vi "DelayTables.vi"() -> ()   [LabVIEW 2022 SP3]
uses:
  <vilib>/Analysis/NI_AALPro.lvlib
  <vilib>/Analysis/NI_AALBase.lvlib
  <vilib>/Analysis/2dsp.llb/1D Cross Correlation (DBL).vi
  <vilib>/Utility/file.llb/Write Delimited Spreadsheet (DBL).vi
  ViewData/-ReadEye/ScaleMethod.ctl
  -AnnularRoutines/ArrayGeometry.ctl
  -AnnularRoutines/TransGeometry.ctl
panel:
  in  "Filter Prams":T1={"low cutoff"=5, "order"=81, "high cutoff"=35}
  in  "Type of Mean":u16(ring) items=["Mean from lines", "Mean just lines", "Poly Mean", "No mean", "Filter"]
  in  "Trans Geometry (mm) out":T2={"Transducer"=0, "Geo Focus"=12.0, "a (radius)"=3.0, "# of rings"=5, "kerf space "=0.1, "Center Freq"=12.0} {"Transducer" items=["6D 12R 40 MHz"=0, "10D 31R 20 MHz"=1, "10D 23R 20 MHz"=2, "6D 23R 40 MHz"=3, "4.5D 10.7R 40 MHz"=4, "9D 23.5R 20 MHz"=5, "9D 25.8R 20MHz"=6, "Enter"=99]}
  in  "index (page)":i32
  in  "d":u8
  out "Blow up of yellow Line 3":dbl[][](graph)
  in  "Case Constant\n(See Context Help)":bool
  out "Waveform Graph":dbl[][](graph)
  in  "Tab Control":enum32{"Page 1", "Page 2", "Page 3"}(tab)
  out "rel set of 6":i32[][](array[numeric])
  in  "Rings mm 2":sgl[](array[numeric])=[0.0, 1.32, 1.42, 1.9, 2.0, 2.36, 2.46, 2.75, 2.85, 3.1]
  out "data delays stacked":i32[][](array[numeric])
  out "rel set of 5":i32[][](array[numeric])
  in  "furthest first?":bool
  out "data delays":i32[][][](array[numeric])
  out "Array":dbl[][](array[numeric]) format="%.2f"
  out "delays abs":dbl[][][](array[numeric]) format="%.2f"
  in  "sampling rate":dbl=1e-09
  in  "focus mm":dbl=12.0
  in  "Rings mm":sgl[](array[numeric])=[0.0, 1.22, 1.32, 1.8, 1.9, 2.26, 2.36, 2.65, 2.75, 3.0]
  in  "focus locations":sgl[](array[numeric])=[9.0, 10.2, 11.0, 12.0, 13.0, 14.0, 15.0]
  in  "sound speed mm/s":dbl=1485000.0
  out "delays":sgl[][](array[numeric]) format="%#_2g"
  in  "delay offset":sgl
  in  "Corr(T)/Thresh(F)":bool
  out "Wire Locations mm":dbl[](array[numeric]) format="%0.2f"
  in  "View Header?":bool
  in  "Axis scaling":bool=TRUE
  out "Scan line peaks":dbl[](array[numeric]) format="%0.2f"
  out "Wire Locations RF":dbl[](array[numeric]) format="%0.2f"
  out "Blow up of yellow Line 2":sgl[](graph)
  in  "new file path":path=path "F:/PVDFXducer/FiveRing/5Ring5/83micH/Wire Phantom/25 micron/WireAugd 1to1.eye"
  out "Blow up of yellow Line":dbl[][](graph)
  out "Raw data":dbl[][](graph)
  in  "Display mode":T4=enum."Log Grey Scale"
  in  "threshold":dbl=20.0 format="%0.2f"
  in  "width":i32=10 min=3
  out "Waveform Graph 2":dbl[][](graph)
  out "Intensity Graph":dbl[][](graph)
  # "time steps to shift relative to zero"
  # "rings"
  # "distances"
  # "Each plane is delays for single focal distance. Negative means subtract zeroes."
  # "receive"
  # "transmit"
  # "relative delays to ring one. Each row is a different focal depth"
  # "Delays relative to ring 1. Starting at furthest ring"
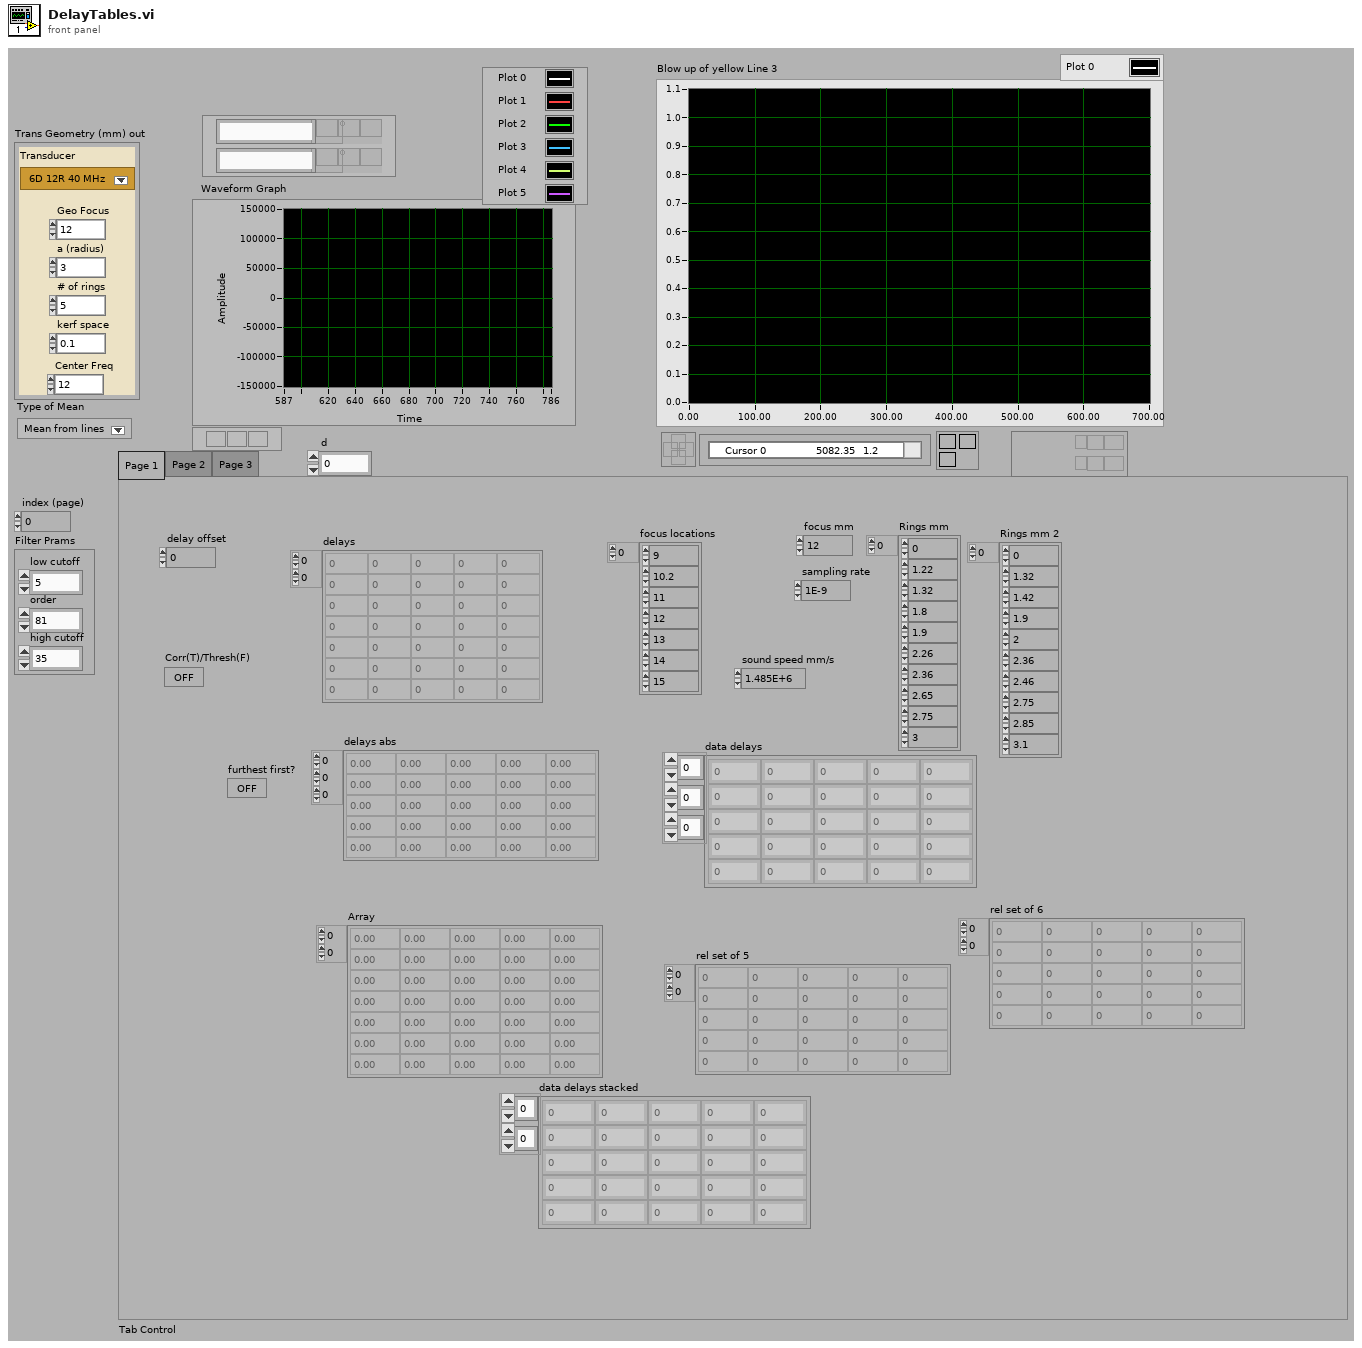
[diagram p1: front panel]
types:
  T1 = cluster{"low cutoff":i32, "order":i32, "high cutoff":i32}
  T2 = typedef "TransGeometry.ctl" = cluster{"Transducer":T3, "Geo Focus":dbl, "a (radius)":dbl, "# of rings":i32, "kerf space ":dbl, "Center Freq":dbl}
  T3 = typedef "ArrayGeometry.ctl" = u16
  T4 = typedef "ScaleMethod.ctl" = enum16{"Linear Abs Grey", "Log Grey Scale", "Linear Color Scale", "dB Scale", "Verasonics Doppler"}
  T5 = typedef "Header.ctl" = cluster{"header info":cluster{"Header":string, "Head length":i16}, "A/D info":cluster{"# rf points per line":u16, "# lines per scan":u16, "sample rate MHz":u16, "# A/D bits":i16, "# bytes per A/D":u16, "TGC Flag":u16, "A/D Type":string}, "Tranducer Info":cluster{"bandwidth":sgl, "center freq":sgl, "start freq":sgl, "ID":i32}, "Scan Info":cluster{"delay":sgl, "pivot distance":sgl, "sector scan angle":sgl, "operator":string, "Scan Mode":string, "location":string}, "Time/Date Info":cluster{"date":string, "time":string}, "RF Info":cluster{"RF file name":string, "RF file att":string, "RF cal file name":string, "RF cal file att":string}, "Patient Info":cluster{"ID":string, "extended ID":string, "age":u16, "sex":string, "previously\nscanned":string, "PSA":sgl, "LOS":u8, "Ethnicty 2":u8, "Race":u8}, "Tissue Type":cluster{"organ":i16, "disease type":i16, "disease location":i16, "IQ_pts":u16, "RcvBuffer":u8, "RcvFrame":u16, "IQBuff":u8, "IQFrame":u16, "IQPage":u8}, "Votage scaling":cluster{"Digitizer (dB)":sgl, "Gain (dB)":sgl, "Atten (dB)":sgl}, "Comment":string, "Misc Info":cluster{"avg num":u16, "c speed":i16, "Div By or SF zones":i16, "XMIT CHS":u8, "RCV CHS":u8, "Xmit angle":sgl}, "Therapy Parameters":cluster{"Theraputic Freq (MHz)":sgl, "Time on (s)":sgl, "Therapy amplitude (mV)":sgl, "Lines Before":u16, "Lines After":u16}, "Scan Settings":cluster{"Energy (uJ or V)":u8, "Damp (Ohm) or Fc":u8, "HP Filt (KHz)":u8, "LP Filt (MHz)":u8, "Gain (db)":u8, "prf (kHz)":sgl, "Distance between\nscan lines (um)":u16, "Distance between\nscan planes (um)":u16, "Scan line gap (um)":sgl, "Scan plane gap (um)":sgl}, "Compression Parameters":cluster{"F1 (MHz)":sgl, "F2 (MHz)":sgl, "% taper":sgl, "duration":sgl}, "Patient Info Xtra":cluster{"First Name":string, "Last Name":string, "Notes":string}, "ROI Box":u16[]}
  T6 = cluster{"Energy (uJ) or V":u8, "Damp (Ohm) or Fc":u8, "HP Filt(KHz) ":u8, "LP Filt (MHz)":u8, "Gain (db)":u8, "prf (kHz)":sgl, "Distance between\nscan lines (mm)":u16, "Distance between\nscan planes (mm)":u16, "Scan line gap (um)":sgl, "Scan plane gap (um)":sgl}
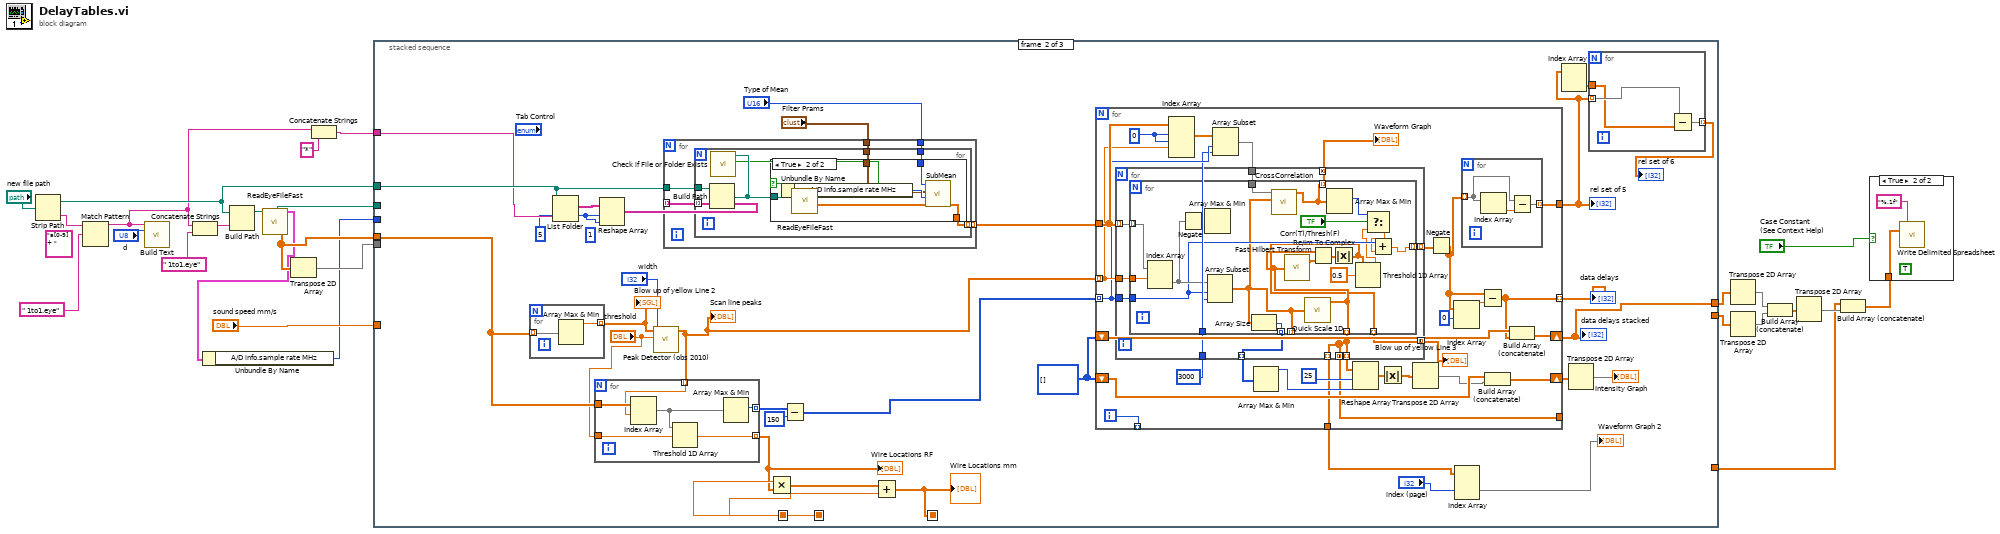
[diagram p0: block diagram]
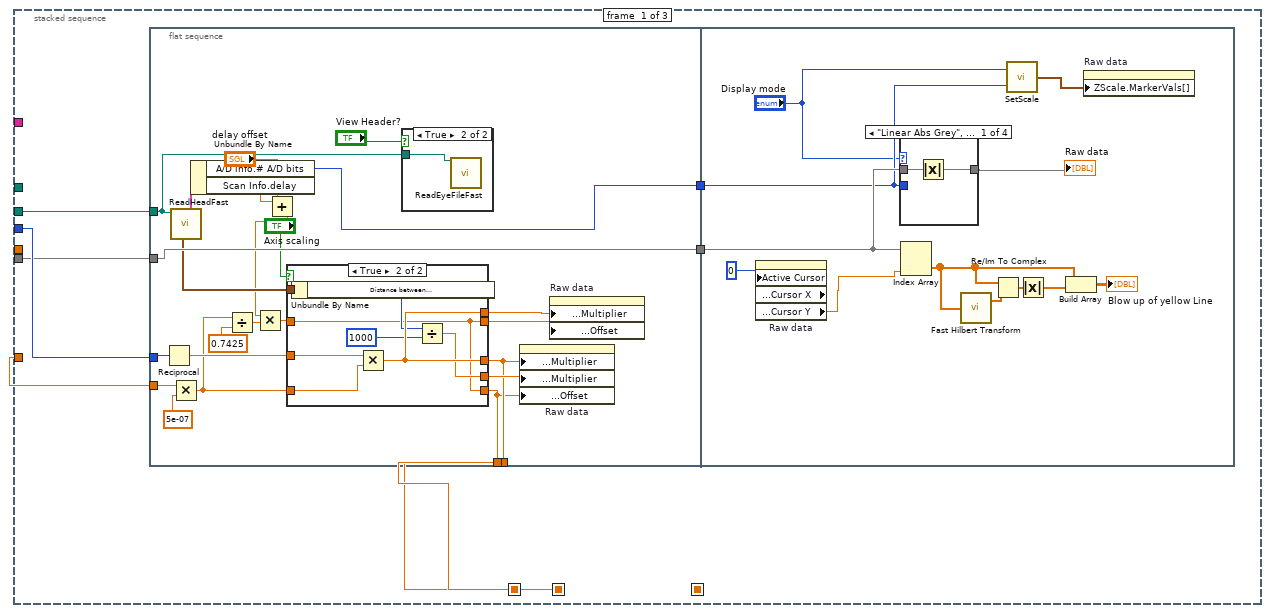
[diagram p3: hidden frame]
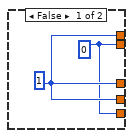
[diagram p5: hidden frame]
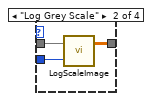
[diagram p6: hidden frame]
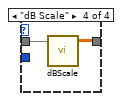
[diagram p8: hidden frame]
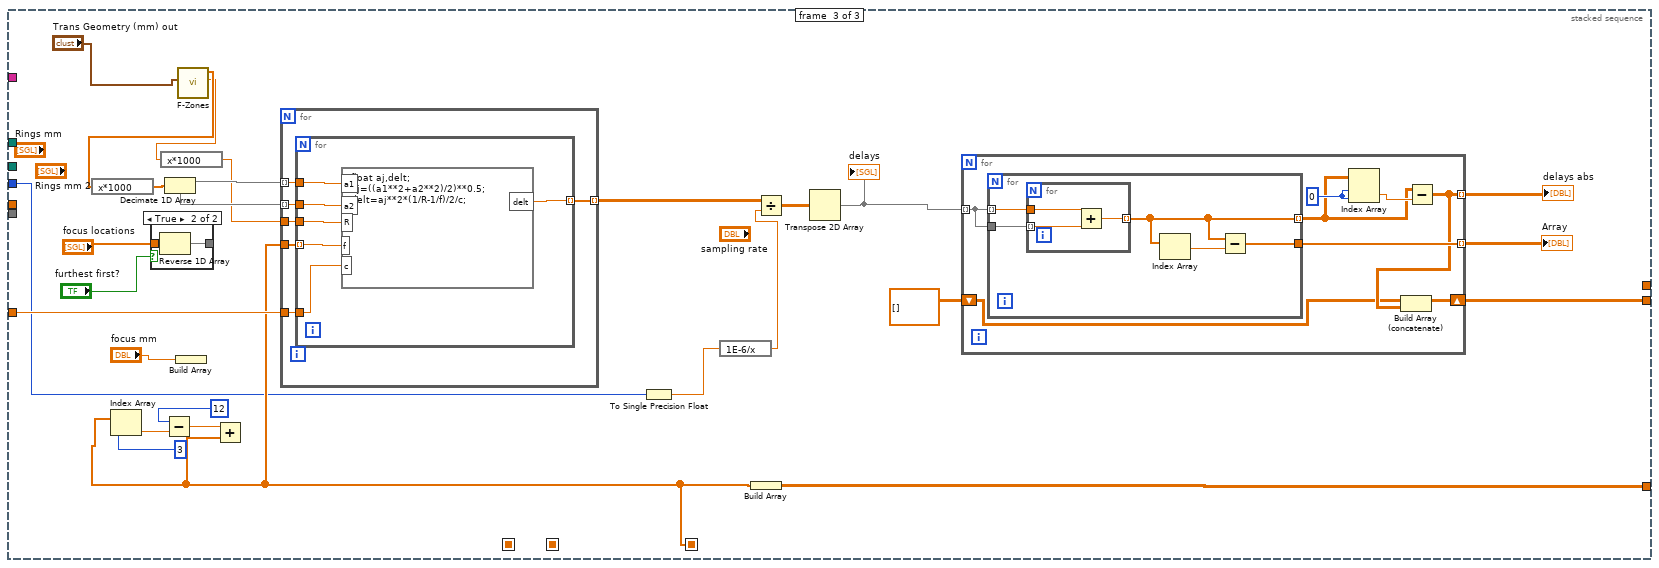
[diagram p10: hidden frame]
diagram:
  (unwired) "a[0-9]+ " ("regular expression")
  n1 = Strip Path(path="new file path") -> (stripped path=w8:path, name=w11:string)
  n2 = Match Pattern(string=w11, regular expression=" 1to1.eye" ("string")) -> (before substring=w1:string)  [unwired: 1 in, 3 out]
  n3 = call "Build Text"("Beginning Text"=w1, "d"="d") -> ()  [unwired: 12 in, 2 out]
  n4 = Concatenate Strings(w1, " 1to1.eye" ("string")) -> (w10:string)
  n5 = Build Path(base path=w8, name or relative path=w10) -> (appended path=w9:path)
  n6 = call "ReadEyeFileFast.vi"("new file path"=w9) -> ("new path out"=w26:path, "2-D data array"=w14:sgl[][], "Header In"=w4:T5)  [unwired: 13 in, 3 out]
  n7 = Unbundle By Name(w4) -> ("A/D info.sample rate MHz"=w3:u16)
  n8 = Transpose 2D Array(2D array=w14) -> (transposed array=w15:sgl[][])
  n9 = Concatenate Strings(w1, "*" ("string")) -> (w5:string)
  n10 = stacked-sequence {
    seq-local: [w30 _ _] -> [_ w116 _]
    seq-local: [w29 _ _] -> [_ w117 _]
    seq-local: [_ w111 _] -> [_ _ w223]
    tunnel: w15 -> [w27 _ _]
    tunnel: w26 -> [w33 _ _]
    tunnel: w3 -> [w32 _ w216]
    tunnel: "sound speed mm/s" -> [w31 _ w233]
    tunnel: [_ _ w227] -> w22
    tunnel: [_ w113 _] -> w23
    tunnel: [_ _ w224] -> w16
    tunnel: w14 -> [_ w109 _]
    tunnel: w8 -> [_ w101 _]
    tunnel: w5 -> [_ w100 _]
    frame #0 {
      n11 = flat-sequence {
        tunnel: w27 -> [w57]
        tunnel: [w57] -> w34
        tunnel: w33 -> [w46]
        tunnel: w32 -> [w52]
        tunnel: w31 -> [w48]
        tunnel: [w45] -> w29
        tunnel: [w44] -> w30
        tunnel: [w38] -> w28
        tunnel: w34 -> [w74]
        tunnel: w28 -> [w71]
        frame #0 {
          n12 = Reciprocal(x=w52) -> (1/x=w51:dbl)
          n13 = call "ReadHeadFast.vi"("new file path"=w46) -> ("Header In"=w39:T5, "Scan Settings (Pulser and Scaping)"=w53:T6)  [unwired: 7 in, 2 out]
          n14 = Multiply(x=w48, y=5e-07) -> (x*y=w42:dbl)
          n15 = Unbundle By Name(w39) -> ("A/D info.# A/D bits"=w38:i16, "Scan Info.delay"=w37:sgl)
          n16 = Divide(x=w42, y=0.7425) -> (x/y=w41:dbl)
          n17 = Add(x=w37, y="delay offset") -> (x+y=w36:sgl)
          n18 = Multiply(x=w36, y=w41) -> (x*y=w40:dbl)
          n19 = case shown="True" "Axis scaling" {
            tunnel: [w60 w68] -> w45
            tunnel: [w60 w68] -> w54
            tunnel: w53 -> [_ w67]
            tunnel: [w60 w64] -> w55
            tunnel: [w59 w63] -> w56
            tunnel: w40 -> [_ w63]
            tunnel: [w59 w63] -> w44
            tunnel: w51 -> [_ w62]
            tunnel: w42 -> [_ w61]
            frame False {
              w59 = 0
              w60 = 1
            }
            frame True {
              n20 = Unbundle By Name(w67) -> ("Distance between\nscan lines (mm)"=w66:u16)
              n21 = Multiply(x=w62, y=w61) -> (x*y=w68:dbl)
              n22 = Divide(x=w66, y=1000) -> (x/y=w64:dbl)
            }
          }
          n23 = case shown="True" "View Header?" {
            tunnel: w46 -> [_ w58]
            frame False {
            }
            frame True {
              n24 = call "ReadEyeFileFast.vi"("new file path"=w58) -> ()  [unwired: 13 in, 6 out]
            }
          }
          n25 = property on="Raw data" class="IntGraph (strict)"("X Scale.Offset and Multiplier:Multiplier"=w45, "Y Scale.Offset and Multiplier:Multiplier"=w55, "X Scale.Offset and Multiplier:Offset"=w44) -> ()  [unwired: 2 in, 2 out]
          n26 = property on="Raw data" class="IntGraph (strict)"("X Scale.Offset and Multiplier:Multiplier"=w54, "X Scale.Offset and Multiplier:Offset"=w56) -> ()  [unwired: 2 in, 2 out]
        }
        frame #1 {
          n27 = property on="Raw data" class="IntGraph (strict)" props=["Active Cursor", "Cursor", "Cursor Position:Cursor X", "Cursor", "Cursor Position:Cursor Y"]("Active Cursor"=u32 0 ("Write Attribute")) -> ("Cursor.Cursor Position:Cursor Y"=w73:dbl)  [unwired: 2 in, 3 out]
          n28 = case shown="\"Linear Abs Grey\", Default" "Display mode" {
            tunnel: [w81 w85 w86 w87] -> w69
            tunnel: w74 -> [w82 w84 w86 w88]
            tunnel: w71 -> [_ w83 _ _]
            frame "Linear Abs Grey", Default {
              n29 = Absolute Value(x=w82) -> (abs(x)=w81:sgl[][])
            }
            frame "Log Grey Scale" {
              n30 = call "LogScaleImage.vi"("A/D bits"=w83, "input array"=w84) -> ("log scale image"=w85:dbl[][])  [unwired: 1 out]
            }
            frame "Linear Color Scale" {
            }
            frame "dB Scale" {
              n31 = call "dBScale.vi"("Data In"=w88) -> ("Data Out"=w87:dbl[][])  [unwired: 4 in]
            }
          }
          "Raw data" <- w69
          n32 = Index Array(array=w74, index (col)=w73) -> (element=w80:sgl[])  [unwired: 1 in]
          n33 = call <vilib>:"Fast Hilbert Transform.vi"("X"=w80) -> ("Hilbert{X}"=w77:dbl[])  [unwired: 1 out]
          n34 = Re/Im To Complex(1:w77, 2:w80) -> (0:w76:cdb[])
          n35 = call "SetScale.vi"("# A/D bits"=w71, "Display mode"="Display mode") -> ("Array"=w72:cluster{dbl, u32}[])
          n36 = Absolute Value(x=w76) -> (abs(x)=w79:dbl[])
          n37 = Build Array(w80, w79) -> (→"Blow up of yellow Line":dbl[][])
          n38 = property on="Raw data" class="IntGraph (strict)"("ZScale.MarkerVals[]"=w72) -> ()  [unwired: 2 in, 2 out]
        }
      }
    }
    frame #1 {
      (unwired) 1
      w99 = 5
      w107 = i32[][] []
      n39 = for {
        tunnel: w109 -> [w212] mode=indexing
        tunnel: [w211] -> w112 mode=indexing
        n40 = Array Max & Min(array=w212) -> (max value=w211:sgl)  [unwired: 3 out]
      }
      "Blow up of yellow Line 2" <- w112
      n41 = List Folder(path=w101, pattern=w100) -> (filenames=w105:string[])  [unwired: 1 in, 4 out]
      n42 = Reshape Array(w105, w99, w99) -> (w106:string[][])
      n43 = call <vilib>:"Peak Detector (obs 2010).vi"("width"="width", "threshold"="threshold", "X"=w112) -> ("Locations"=w110:dbl[])  [unwired: 4 in, 4 out]
      "Scan line peaks" <- w110
      n44 = for {
        tunnel: [w209] -> w114 mode=indexing
        tunnel: w109 -> [w210]
        tunnel: w110 -> [w206] mode=indexing
        tunnel: [w207] -> w115 mode=indexing
        tunnel: "threshold" -> [w205]
        n45 = Index Array(array=w210, index (row)=w206) -> (element=w208:sgl[])  [unwired: 1 in]
        n46 = Threshold 1D Array(2:w205, 3:w208) -> (0:w207:sgl)  [unwired: 1 out]
        n47 = Array Max & Min(array=w208) -> (max index (indices)=w209:i32)  [unwired: 3 out]
      }
      "Wire Locations RF" <- w115
      n48 = for {
        tunnel: [w128] -> w104 mode=indexing
        tunnel: w106 -> [w127] mode=indexing
        tunnel: w101 -> [w126]
        tunnel: "Type of Mean" -> [w125]
        tunnel: "Filter Prams" -> [w124]
        n49 = for {
          tunnel: [w131] -> w128 mode=indexing
          tunnel: w127 -> [w135] mode=indexing
          tunnel: w126 -> [w134]
          tunnel: w125 -> [w130]
          tunnel: w124 -> [w129]
          n50 = Build Path(base path=w134, name or relative path=w135) -> (appended path=w133:path)
          n51 = call <vilib>:"Check if File or Folder Exists.vi"("path"=w133) -> ("file or folder exists?"=w132:bool)  [unwired: 8 in, 2 out]
          n52 = case shown="True" w132 {
            tunnel: w133 -> [_ w142]
            tunnel: [_ w140] -> w131
            tunnel: w130 -> [_ w139]
            tunnel: w129 -> [_ w136]
            frame False {
            }
            frame True {
              n53 = call "ReadEyeFileFast.vi"("new file path"=w142) -> ("2-D data array"=w141:sgl[][], "Header In"=w138:T5)  [unwired: 13 in, 4 out]
              n54 = Unbundle By Name(w138) -> ("A/D info.sample rate MHz"=w137:u16)
              n55 = call "SubMean.vi"("Scan Data In"=w141, "Samp Rate (MHz)"=w137, "Filter Prams"=w136, "Type of Mean"=w139) -> ("Array"=w140:dbl[][])  [unwired: 1 in, 2 out]
            }
          }
        }
      }
      n56 = Multiply(x=w117, y=w115) -> (x*y=w118:dbl[])
      n57 = Subtract(x=w114, y=150) -> (x-y=w119:i32[])
      n58 = Add(x=w118, y=w116) -> (x+y=w111:dbl[])
      "Wire Locations mm" <- w111
      n59 = for {
        tunnel: w110 -> [w150] mode=indexing
        tunnel: [w162] -> w108 mode=indexing
        tunnel: w119 -> [w149] mode=indexing
        shift-right: [w166] -> w103
        shift-left: w107 -> [w161]
        shift-right: [w164] -> w113
        shift-left: w107 -> [w163]
        tunnel: w104 -> [w157]
        tunnel: [w158] -> w95
        tunnel: [w152] -> _ mode=indexing
        tunnel: [w145] -> _
        tunnel: [w143] -> w98
        i -> [w152]
        w151 = 0
        w148 = 3000
        w170 = 0
        n60 = Index Array(array=w157, index (dim 0)=w151, index (dim 1)=w151, index (dim 2)=w150) -> (element=w155:dbl[])  [unwired: 1 in]
        n61 = Array Subset(array=w155, index=w149, length=w148) -> (w156:dbl[])
        n62 = for {
          tunnel: [w175] -> w171 mode=indexing
          tunnel: [w184] -> w168 mode=indexing
          tunnel: w150 -> [w183]
          tunnel: w148 -> [w182]
          tunnel: w149 -> [w181]
          tunnel: w157 -> [w180] mode=indexing
          tunnel: w156 -> [w179]
          tunnel: [w178] -> w154 mode=indexing
          tunnel: [w177] -> w147 mode=concatenating
          tunnel: [w175] -> w145 mode=concatenating
          tunnel: [w176] -> w144 mode=concatenating
          tunnel: [w175] -> w143 mode=indexing
          n63 = for {
            tunnel: [w194] -> w184 mode=indexing
            tunnel: [w190] -> w175 mode=indexing
            tunnel: w183 -> [w197]
            tunnel: w182 -> [w195]
            tunnel: w181 -> [w196]
            tunnel: w180 -> [w201] mode=indexing
            tunnel: w179 -> [w199]
            tunnel: [w198] -> w178 mode=indexing
            tunnel: [w189] -> w177 mode=indexing
            tunnel: [w193] -> _ mode=indexing
            tunnel: [w191] -> w176 mode=indexing
            n64 = Index Array(array=w201, index (row)=w197) -> (element=w200:dbl[])  [unwired: 1 in]
            n65 = Negate(x=w200) -> (-x=w192:dbl[])
            n66 = Array Max & Min(array=w192) -> ()  [unwired: 4 out]
            n67 = Array Subset(array=w200, index=w196, length=w195) -> (w193:dbl[])
            n68 = Array Size(array=w193) -> (size(s)=w198:i32)
            n69 = call-poly <vilib>:"CrossCorrelation.vi"("Y"=w193, "X"=w199) -> ("Rxy"=w191:dbl[])  [unwired: 2 in, 7 out]
            n70 = call <vilib>:"Quick Scale 1D.vi"("X"=w193) -> ("Y[i]=X[i]/Max|X|"=w190:dbl[])  [unwired: 2 out]
            n71 = call <vilib>:"Fast Hilbert Transform.vi"("X"=w190) -> ("Hilbert{X}"=w202:dbl[])  [unwired: 1 out]
            n72 = Re/Im To Complex(1:w202, 2:w190) -> (0:w203:cdb[])
            n73 = Array Max & Min(array=w191) -> (max index (indices)=w188:i32)  [unwired: 3 out]
            n74 = Absolute Value(x=w203) -> (abs(x)=w189:dbl[])
            n75 = Threshold 1D Array(2:0.5, 3:w189) -> (0:w187:dbl)  [unwired: 1 out]
            n76 = Select(t=w188, s="Corr(T)/Thresh(F)", f=w187) -> (s? t:f=w186:dbl)
            n77 = Add(x=w196, y=w186) -> (x+y=w194:dbl)
          }
        }
        "Blow up of yellow Line 3" <- w147
        "Waveform Graph" <- w144
        n78 = Array Max & Min(array=w154) -> (max value=w153:i32)  [unwired: 3 out]
        n79 = Reshape Array(w171, 25, w153) -> (w146:dbl[][])
        n80 = Absolute Value(x=w146) -> (abs(x)=w165:dbl[][])
        n81 = Transpose 2D Array(2D array=w165) -> (transposed array=w160:dbl[][])
        n82 = Negate(x=w168) -> (-x=w159:dbl[][])
        n83 = Index Array(array=w159, index (row)=w170, index (col)=w170) -> (element=w169:dbl)
        n84 = for {
          tunnel: w159 -> [w173] mode=indexing
          tunnel: [w172] -> w158 mode=indexing
          n85 = Index Array(array=w173) -> (element=w174:dbl)  [unwired: 1 in]
          n86 = Subtract(x=w173, y=w174) -> (x-y=w172:dbl[])
        }
        n87 = Subtract(x=w159, y=w169) -> (x-y=w162:dbl[][])
        n88 = Build Array (concatenate)(w161, w160) -> (w166:dbl[][])
        n89 = Build Array (concatenate)(w163, w162) -> (w164:dbl[][])
      }
      "data delays" <- w108
      "data delays stacked" <- w113
      "rel set of 5" <- w95
      n90 = Index Array(array=w98, index (dim 1)="index (page)") -> (element=→"Waveform Graph 2":dbl[][])  [unwired: 2 in]
      n91 = Index Array(array=w95) -> (element=w94:dbl[])  [unwired: 2 in]
      n92 = Transpose 2D Array(2D array=w103) -> (transposed array=→"Intensity Graph":dbl[][])
      n93 = for {
        tunnel: w95 -> [w123] mode=indexing
        tunnel: [w122] -> w93 mode=indexing
        tunnel: w94 -> [w121]
        n94 = Subtract(x=w123, y=w121) -> (x-y=w122:dbl[])
      }
      "rel set of 6" <- w93
    }
    frame #2 {
      n95 = Index Array(array=w223, index=3) -> (element=w229:dbl)
      n96 = case shown="True" "furthest first?" {
        tunnel: "focus locations" -> [w240 w242]
        tunnel: [w240 w241] -> _
        frame False {
        }
        frame True {
          n97 = Reverse 1D Array(array=w242) -> (reversed array=w241:sgl[])
        }
      }
      n98 = Subtract(x=12, y=w229) -> (x-y=w231:dbl)
      n99 = Build Array("focus mm") -> ()  [unwired: 1 out]
      n100 = call "F-Zones.vi"("Trans Geometry (mm)"="Trans Geometry (mm) out") -> ("ROC (m)"=w220:dbl, "annuli rad (m)"=w222:dbl[])  [unwired: 7 in, 2 out]
      n101 = expression code="x*1000"(w222) -> (w221:dbl[])
      n102 = expression code="x*1000"(w220) -> (w219:dbl)
      n103 = Decimate 1D Array(w221) -> (w238:dbl[], w237:dbl[])
      n104 = Add(x=w231, y=w223) -> ()  [unwired: 1 out]
      n105 = for {
        tunnel: w233 -> [w248]
        tunnel: w223 -> [w247]
        tunnel: w238 -> [w246] mode=indexing
        tunnel: w237 -> [w245] mode=indexing
        tunnel: [w244] -> w236 mode=indexing
        tunnel: w219 -> [w243]
        n106 = for {
          tunnel: w247 -> [w254] mode=indexing
          tunnel: w248 -> [w253]
          tunnel: w246 -> [w252]
          tunnel: w245 -> [w251]
          tunnel: [w250] -> w244 mode=indexing
          tunnel: w243 -> [w249]
          n107 = formula code="float aj,delt;\naj=((a1**2+a2**2)/2)**0.5;\ndelt=aj**2*(1/R-1/f)/2/c;"("a1"=w252, "a2"=w251, "f"=w254, "c"=w253, "R"=w249) -> ("delt"=w250:dbl)
        }
      }
      n108 = To Single Precision Float(number=w216) -> (single precision float=w215:sgl)
      n109 = expression code="1E-6/x"(w215) -> (w213:sgl)
      n110 = Build Array(w223) -> (w224:dbl[][])
      n111 = Divide(x=w236, y=w213) -> (x/y=w214:dbl[][])
      n112 = Transpose 2D Array(2D array=w214) -> (transposed array=w235:dbl[][])
      "delays" <- w235
      n113 = for {
        tunnel: w235 -> [w262] mode=indexing
        tunnel: [w257] -> w226 mode=indexing
        tunnel: [w261] -> w225 mode=indexing
        shift-right: [w255] -> w227
        shift-left: dbl[][] [] -> [w256]
        w260 = 0
        n114 = for {
          tunnel: w262 -> [w266] mode=indexing
          tunnel: w262 -> [w267]
          tunnel: [w263] -> w258 mode=indexing
          tunnel: [w264] -> w261
          n115 = for {
            tunnel: w267 -> [w270] mode=indexing
            tunnel: w266 -> [w269]
            tunnel: [w268] -> w263 mode=indexing
            n116 = Add(x=w269, y=w270) -> (x+y=w268:dbl)
          }
          n117 = Index Array(array=w263) -> (element=w265:dbl)  [unwired: 1 in]
          n118 = Subtract(x=w263, y=w265) -> (x-y=w264:dbl[])
        }
        n119 = Index Array(array=w258, index (row)=w260, index (col)=w260) -> (element=w259:dbl)
        n120 = Subtract(x=w258, y=w259) -> (x-y=w257:dbl[][])
        n121 = Build Array (concatenate)(w256, w257) -> (w255:dbl[][])
      }
      "delays abs" <- w226
      "Array" <- w225
    }
  }
  n122 = Transpose 2D Array(2D array=w23) -> (transposed array=w21:dbl[][])
  n123 = Transpose 2D Array(2D array=w22) -> (transposed array=w20:dbl[][])
  n124 = Build Array (concatenate)(w21, w20) -> (w19:dbl[][])
  n125 = Transpose 2D Array(2D array=w19) -> (transposed array=w18:dbl[][])
  n126 = Build Array (concatenate)(w16, w18) -> (w17:dbl[][])
  n127 = case shown="True" "Case Constant\n(See Context Help)" {
    tunnel: w17 -> [_ w272]
    frame False {
    }
    frame True {
      (unwired) TRUE
      n128 = call-poly <vilib>:"Write Delimited Spreadsheet.vi"("format (%.3f)"="%.1f", "2D data"=w272) -> ()  [unwired: 12 in, 2 out]
    }
  }
